vi "Servo MSMT Set RF Power.vi"(8 "error in (no error)":errorcluster, 10 "Step In":refnum<k7>, 11 "Input Power Measurement in":refnum<class "Input Power Measurement.lvclass">) -> (0 "error out":errorcluster, 2 "Step Out":refnum<k7>, 3 "Input Power Measurement out":refnum<class "Input Power Measurement.lvclass">)   [LabVIEW 2018, in "Input Power Measurement.lvlib" / "Input Power Measurement.lvclass"]
uses:
  Input Power Measurement.lvclass
  C:/Sequence Automation/Plugins/Measurement Interface.lvlibp/Measurement Interface.lvclass
  C:/Sequence Automation/Plugins/Measurements/Servo MSMT.lvlibp/Servo MSMT.lvclass
  Plugins/Measurement Interface.lvlibp/Private Methods/Measurement Parameters/Read Measurement Parameters.vi
  Plugins/Measurement Interface.lvlibp/Private Methods/Test Group Manager/Read Test Group Manager.vi
  <vilib>/Utility/error.llb/Error Cluster From Error Code.vi
  Plugins/String Database.lvlibp/String Database.lvclass
  Plugins/Test Group Manager.lvlibp/Test Group Manager.lvclass
  <vilib>/ErrorRing/Error Ring.xnode
  Plugins/Measurements/Servo MSMT.lvlibp/Servo MSMT.lvclass
  Plugins/TestStand API Tools (TSAT).lvlibp/Step Actions/TSAT Step Actions.lvlib
  Plugins/Test Group Manager.lvlibp/Includes/Test Group/Test Group.lvclass
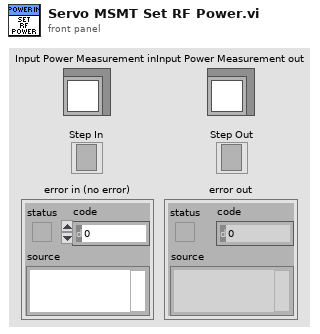
[diagram p1: front panel]
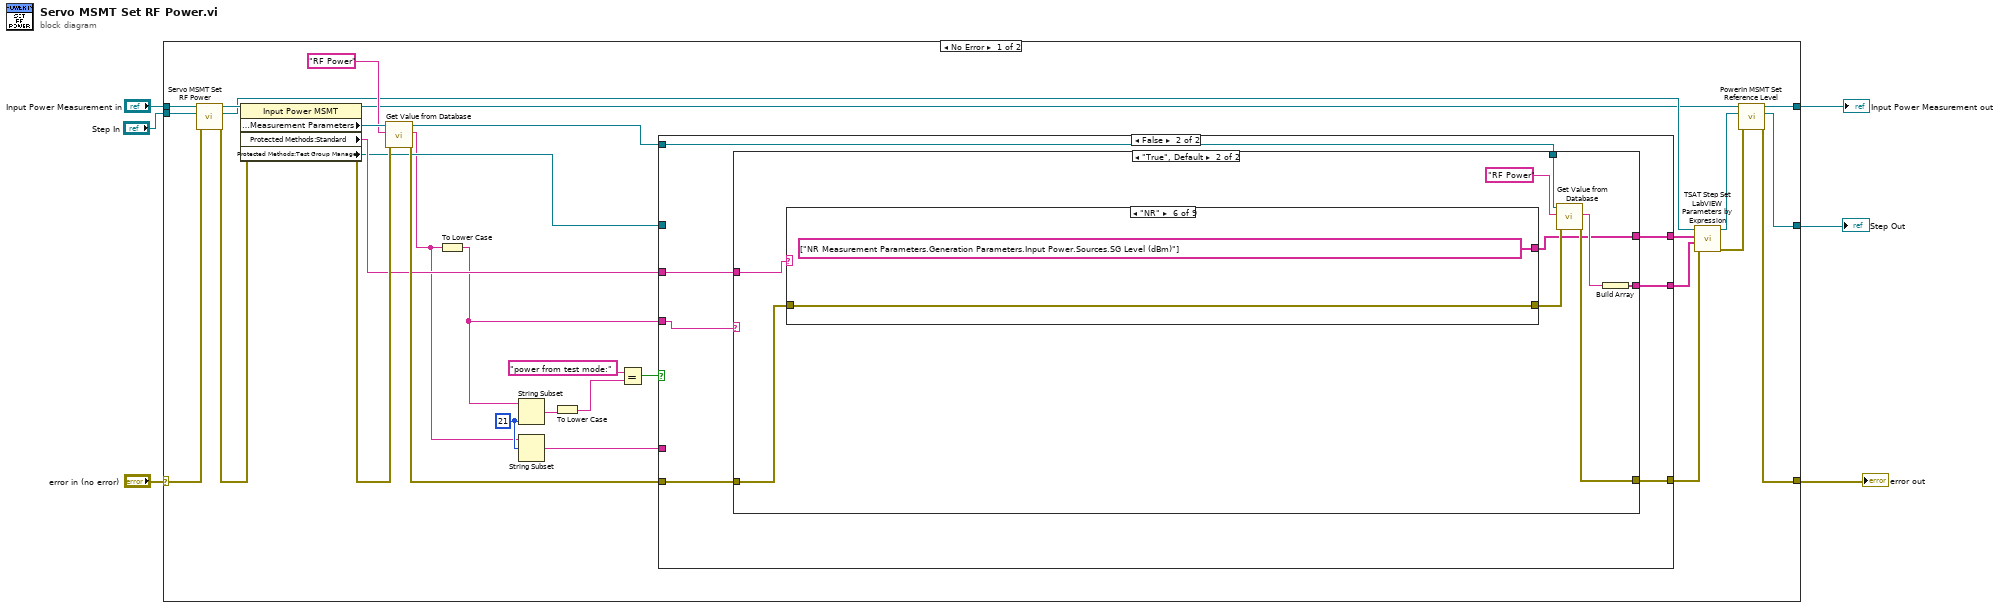
[diagram p0: block diagram]
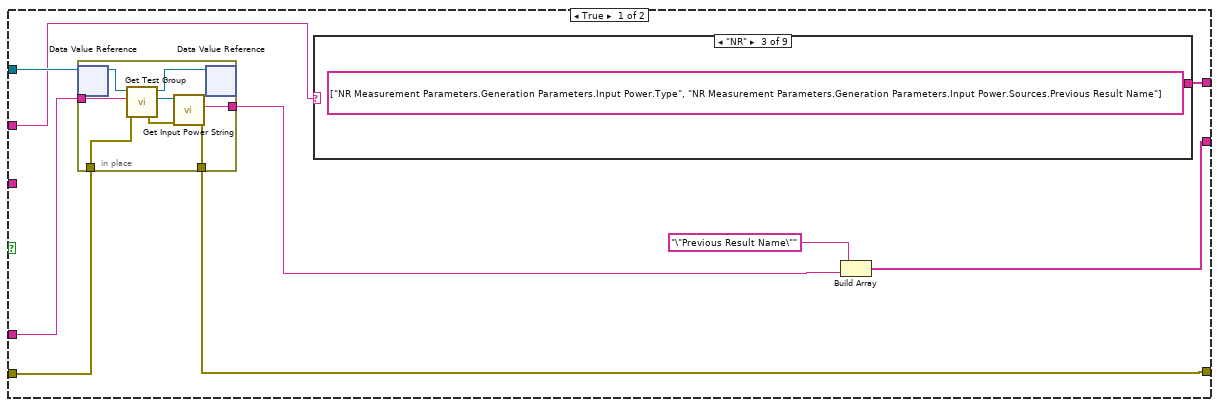
[diagram p2: hidden frame]
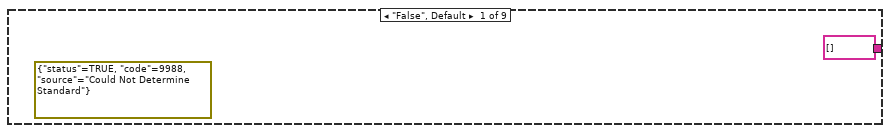
[diagram p3: hidden frame]
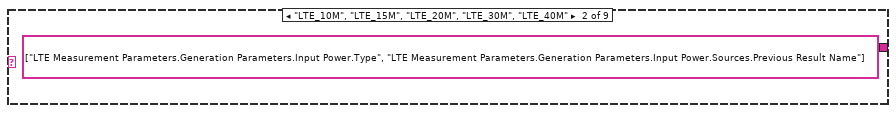
[diagram p4: hidden frame]
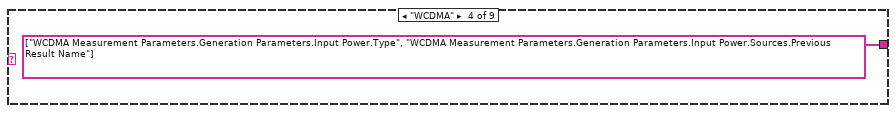
[diagram p5: hidden frame]
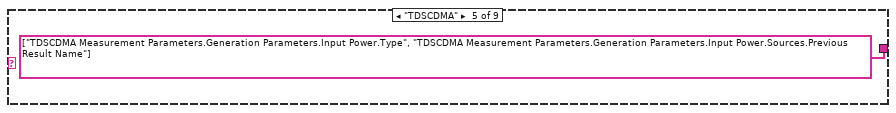
[diagram p6: hidden frame]
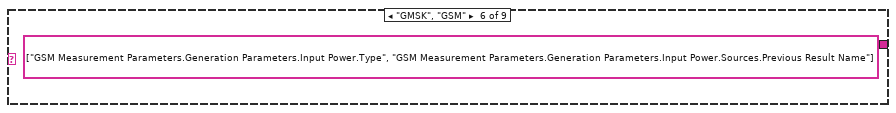
[diagram p7: hidden frame]
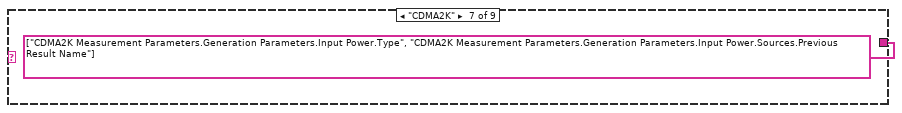
[diagram p8: hidden frame]
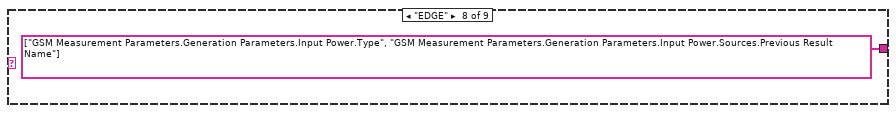
[diagram p9: hidden frame]
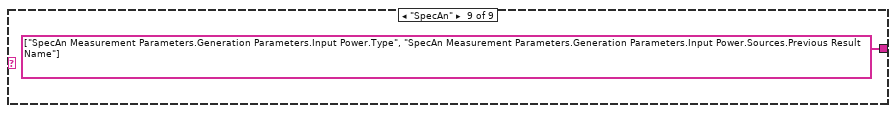
[diagram p10: hidden frame]
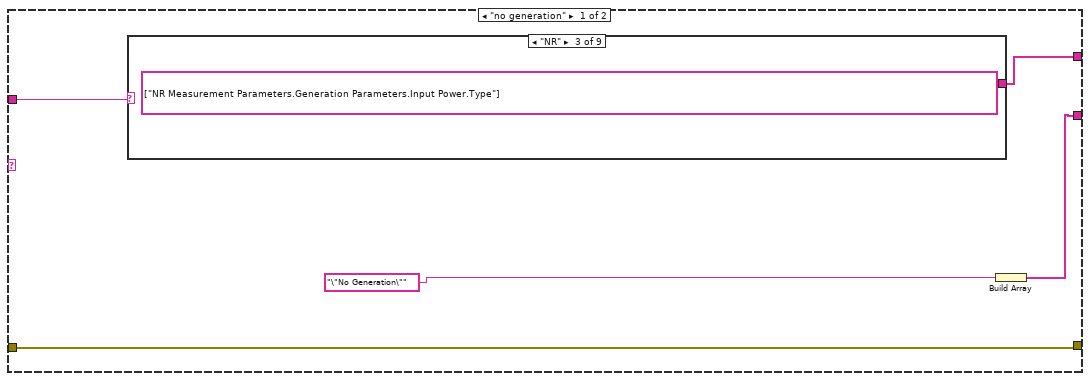
[diagram p11: hidden frame]
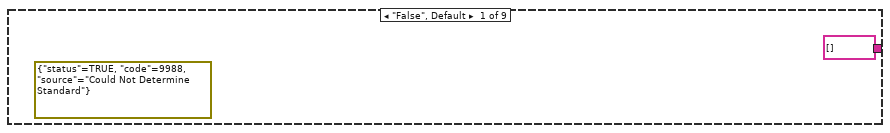
[diagram p12: hidden frame]
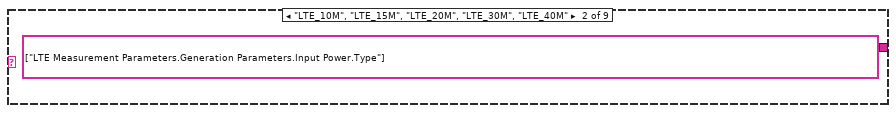
[diagram p13: hidden frame]
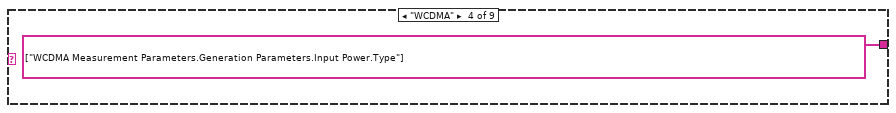
[diagram p14: hidden frame]
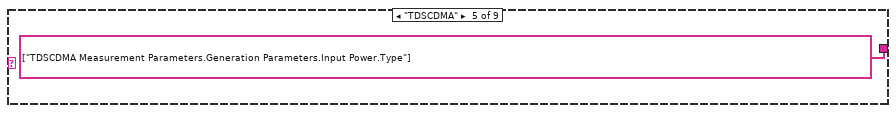
[diagram p15: hidden frame]
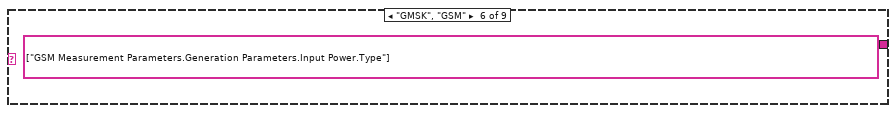
[diagram p16: hidden frame]
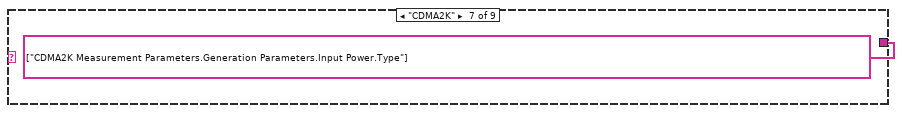
[diagram p17: hidden frame]
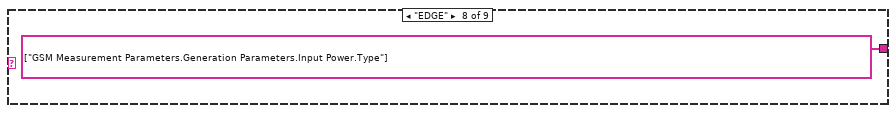
[diagram p18: hidden frame]
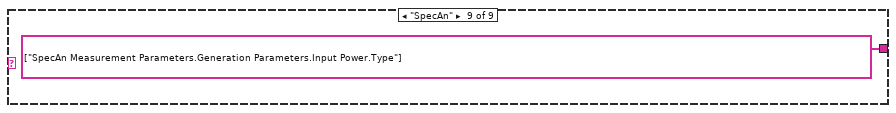
[diagram p19: hidden frame]
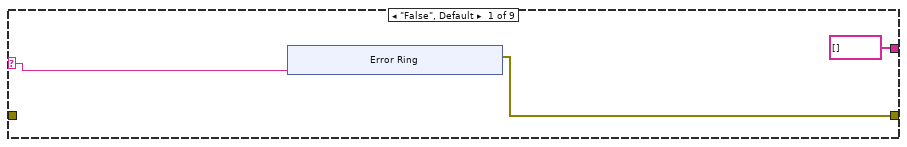
[diagram p20: hidden frame]
diagram:
  n1 = case shown="No Error" "error in (no error)" {
    selector: "error in (no error)" -> [w33 w119]
    tunnel: [w12 w119] -> w5
    tunnel: [w10 w121] -> w4
    tunnel: [w8 w120] -> w3
    tunnel: "Input Power Measurement in" -> [w25 w121]
    tunnel: "Step In" -> [w23 w120]
    frame No Error {
      w15 = 21 ("length (rest)")
      n2 = call-parent "Servo MSMT Set RF Power.vi"("error in (no error)"=w33, "Step In"=w23, "Servo MSMT in"=w25) -> ("error out"=w26:errorcluster, "Step Out"=w22:refnum<k7>, "Servo MSMT out"=w24:refnum<class "Input Power Measurement.lvclass">)  [unwired: 6 in]
      n3 = property class="Input Power MSMT"(reference=w24, error in=w26) -> (reference out=w11:refnum<class "Input Power Measurement.lvclass">, error out=w30:errorcluster, "Protected Methods:Measurement Parameters"=w31:refnum<class "String Database.lvclass">, "Protected Methods:Standard"=w21:string, "Protected Methods:Test Group Manager"=w17:refnum<data-value>)
      n4 = call "Get Value from Database.vi"("error in (no error)"=w30, "Entry Name"="RF Power", "Message in"=w31) -> ("error out"=w29:errorcluster, "Entry Value"=w13:string, "Message out"=w27:refnum<class "String Database.lvclass">)  [unwired: 5 in, 1 out]
      n5 = To Lower Case(string=w13) -> (all lower case string=w7:string)
      n6 = String Subset(string=w7, length (rest)=w15) -> (substring=w16:string)  [unwired: 1 in]
      n7 = String Subset(string=w13, offset (0)=w15) -> (substring=w14:string)  [unwired: 1 in]
      n8 = To Lower Case(string=w16) -> (all lower case string=w19:string)
      n9 = Equal?(x="power from test mode:" ("regular expression"), y=w19) -> (x = y?=w18:bool)
      n10 = case shown="False" w18 {
        tunnel: [w43 w68] -> w36
        tunnel: [w42 w67] -> w35
        tunnel: [w44 w66] -> w34
        tunnel: w27 -> [_ w69]
        tunnel: w29 -> [w45 w65]
        tunnel: w21 -> [w37 w64]
        tunnel: w17 -> [w38 _]
        tunnel: w14 -> [w39 _]
        tunnel: w7 -> [_ w63]
        frame True {
          n11 = in-place {
            in-place-border: w45 -> [w53]
            in-place-border: [w52] -> w43
            in-place-border: [w51] -> w40
            in-place-border: w39 -> [w48]
            n12 = in-place-dvr #1(w38) -> (w47:refnum<class "Test Group Manager.lvclass">)  [unwired: 1 out]
            n13 = call "Get Test Group.vi"("error in (no error)"=w53, "Test Group Name"=w48, "Test Group Manager in"=w47) -> ("error out"=w50:errorcluster, "Test Group In"=w49:refnum<data-value>, "Test Group Manager out"=w46:refnum<class "Test Group Manager.lvclass">)  [unwired: 6 in]
            n14 = call "Get Input Power String.vi"("error in (no error)"=w50, "Test Group In"=w49) -> ("error out"=w52:errorcluster, "Input Power"=w51:string)  [unwired: 7 in, 1 out]
            n15 = in-place-dvr #1(w46) -> ()  [unwired: 2 out]
          }
          n16 = case shown="\"NR\"" w37 {
            tunnel: [string[] [] string[] ["LTE Measurement Parameters.Generation Parameters.Input Power.Type", "LTE Measurement Parameters.Generation Parameters.Input Power.Sources.Previous Result Name"] string[] ["NR Measurement Parameters.Generation Parameters.Input Power.Type", "NR Measurement Parameters.Generation Parameters.Input Power.Sources.Previous Result Name"] string[] ["WCDMA Measurement Parameters.Generation Parameters.Input Power.Type", "WCDMA Measurement Parameters.Generation Parameters.Input Power.Sources.Previous Result Name"] string[] ["TDSCDMA Measurement Parameters.Generation Parameters.Input Power.Type", "TDSCDMA Measurement Parameters.Generation Parameters.Input Power.Sources.Previous Result Name"] string[] ["GSM Measurement Parameters.Generation Parameters.Input Power.Type", "GSM Measurement Parameters.Generation Parameters.Input Power.Sources.Previous Result Name"] string[] ["CDMA2K Measurement Parameters.Generation Parameters.Input Power.Type", "CDMA2K Measurement Parameters.Generation Parameters.Input Power.Sources.Previous Result Name"] string[] ["GSM Measurement Parameters.Generation Parameters.Input Power.Type", "GSM Measurement Parameters.Generation Parameters.Input Power.Sources.Previous Result Name"] string[] ["SpecAn Measurement Parameters.Generation Parameters.Input Power.Type", "SpecAn Measurement Parameters.Generation Parameters.Input Power.Sources.Previous Result Name"]] -> w44
            frame "False", Default {
              (unwired) errorcluster {"status"=TRUE, "code"=9988, "source"="Could Not Determine Standard"} ("error out")
            }
            frame "LTE_10M", "LTE_15M", "LTE_20M", "LTE_30M", "LTE_40M" {
            }
            frame "NR" {
            }
            frame "WCDMA" {
            }
            frame "TDSCDMA" {
            }
            frame "GMSK", "GSM" {
            }
            frame "CDMA2K" {
            }
            frame "EDGE" {
            }
            frame "SpecAn" {
            }
          }
          n17 = Build Array("\"Previous Result Name\"", w40) -> (w42:string[])
        }
        frame False {
          n18 = case shown="\"True\", Default" w63 {
            tunnel: w69 -> [_ w92]
            tunnel: [w70 w89] -> w68
            tunnel: [w72 w87] -> w67
            tunnel: [w71 w86] -> w66
            tunnel: w65 -> [w70 w85]
            tunnel: w64 -> [w74 w84]
            frame "no generation" {
              n19 = case shown="\"NR\"" w74 {
                tunnel: [string[] [] string[] ["LTE Measurement Parameters.Generation Parameters.Input Power.Type"] string[] ["NR Measurement Parameters.Generation Parameters.Input Power.Type"] string[] ["WCDMA Measurement Parameters.Generation Parameters.Input Power.Type"] string[] ["TDSCDMA Measurement Parameters.Generation Parameters.Input Power.Type"] string[] ["GSM Measurement Parameters.Generation Parameters.Input Power.Type"] string[] ["CDMA2K Measurement Parameters.Generation Parameters.Input Power.Type"] string[] ["GSM Measurement Parameters.Generation Parameters.Input Power.Type"] string[] ["SpecAn Measurement Parameters.Generation Parameters.Input Power.Type"]] -> w71
                frame "False", Default {
                  (unwired) errorcluster {"status"=TRUE, "code"=9988, "source"="Could Not Determine Standard"} ("error out")
                }
                frame "LTE_10M", "LTE_15M", "LTE_20M", "LTE_30M", "LTE_40M" {
                }
                frame "NR" {
                }
                frame "WCDMA" {
                }
                frame "TDSCDMA" {
                }
                frame "GMSK", "GSM" {
                }
                frame "CDMA2K" {
                }
                frame "EDGE" {
                }
                frame "SpecAn" {
                }
              }
              n20 = Build Array("\"No Generation\"") -> (w72:string[])
            }
            frame "True", Default {
              n21 = case shown="\"NR\"" w84 {
                selector: w84 -> [w94 _ _ _ _ _ _ _ _]
                tunnel: [w93 w104 w106 w108 w110 w112 w113 w116 w118] -> w90
                tunnel: w85 -> [_ w104 w106 w108 w110 w112 w113 w116 w118]
                tunnel: [string[] [] string[] ["CDMA2K Measurement Parameters.Generation Parameters.Input Power.Sources.SG Level (dBm)"] string[] ["GSM Measurement Parameters.Generation Parameters.Input Power.Sources.SG Level (dBm)"] string[] ["GSM Measurement Parameters.Generation Parameters.Input Power.Sources.SG Level (dBm)"] string[] ["LTE Measurement Parameters.Generation Parameters.Input Power.Sources.SG Level (dBm)"] string[] ["NR Measurement Parameters.Generation Parameters.Input Power.Sources.SG Level (dBm)"] string[] ["SpecAn Measurement Parameters.Generation Parameters.Input Power.Sources.SG Level (dBm)"] string[] ["TDSCDMA Measurement Parameters.Generation Parameters.Input Power.Sources.SG Level (dBm)"] string[] ["WCDMA Measurement Parameters.Generation Parameters.Input Power.Sources.SG Level (dBm)"]] -> w86
                frame "False", Default {
                  n22 = xnode "Error Ring"("parameter 0"=w94) -> ("error out"=w93:errorcluster)
                }
                frame "CDMA2K" {
                }
                frame "EDGE" {
                }
                frame "GMSK", "GSM" {
                }
                frame "LTE", "LTE_10M", "LTE_15M", "LTE_20M", "LTE_30M", "LTE_40M" {
                }
                frame "NR" {
                }
                frame "SpecAn" {
                }
                frame "TDSCDMA" {
                }
                frame "WCDMA" {
                }
              }
              n23 = call "Get Value from Database.vi"("error in (no error)"=w90, "Entry Name"="RF Power", "Message in"=w92) -> ("error out"=w89:errorcluster, "Entry Value"=w88:string)  [unwired: 5 in, 2 out]
              n24 = Build Array(w88) -> (w87:string[])
            }
          }
        }
      }
      n25 = call "TSAT Step Set LabVIEW Parameters by Expression.vi"("Error In"=w36, "Value Expressions"=w35, "Parameters to Set"=w34, "Step In"=w22) -> ("Error Out"=w32:errorcluster, "Step Out"=w9:refnum<k7>)  [unwired: 6 in]
      n26 = call "PowerIn MSMT Set Reference Level.vi"("error in (no error)"=w32, "Step In"=w9, "Input Power MSMT in"=w11) -> ("error out"=w12:errorcluster, "Step Out"=w8:refnum<k7>, "Input Power MSMT out"=w10:refnum<class "Input Power Measurement.lvclass">)  [unwired: 6 in]
    }
    frame Error {
    }
  }
  "error out" <- w5
  "Input Power Measurement out" <- w4
  "Step Out" <- w3
